vi "Get Channel Blocks.vi"(11 "Transfer Configuration in":refnum<class "Transfer Configuration.lvclass">) -> (2 "channel blocks":T1[](array[typedef]) {"buffer offset" format="%d bytes"}, 3 "Transfer Configuration out":refnum<class "Transfer Configuration.lvclass">)   [LabVIEW 2017, in "Data Sharing Framework Engine.lvlib" / "Transfer Configuration.lvclass"]
uses:
  Transfer Configuration.lvclass
  old/dsf core/Source/Shared/Typedefs/DSF Runtime Channel Block.ctl
  old/dsf core/Source/DSF Configuration API/1.0.0/Public/Controls/DSF Data Type.ctl
  Transfer Configuration.lvclass/Transfer Configuration.ctl
  Data Sharing Framework Engine.lvlib
  old/dsf core/Source/DSF Configuration API/1.0.0/DSF Configuration API.lvlib
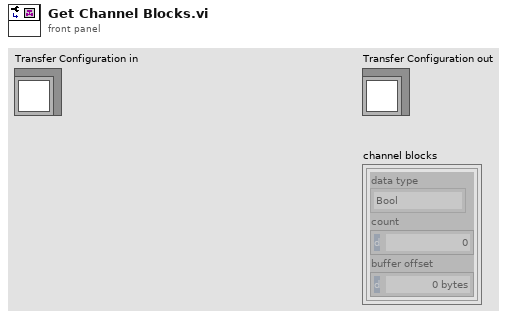
[diagram p1: front panel]
types:
  T1 = typedef "Data Sharing Framework Engine.lvlib/DSF Runtime Channel Block.ctl" = cluster{"data type":T2, "count":u64, "buffer offset":u64}
  T2 = typedef "DSF Configuration API.lvlib/DSF Data Type.ctl" = enum8{"Bool", "SGL", "DBL", "I8", "I16", "I32", "I64", "U8", "U16", "U32", "U64"}
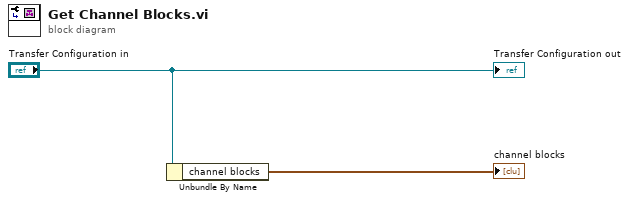
[diagram p0: block diagram]
diagram:
  n1 = Unbundle By Name("Transfer Configuration in") -> ("channel blocks"=→"channel blocks":T1[])
  "Transfer Configuration out" <- "Transfer Configuration in"
